vi "motor follow.vi"() -> ()   [LabVIEW 2009]
uses:
  <vilib>/NXT/Block Support/NXT_OutputPort.ctl
panel:
  in  "coeffecients":cluster{"P":dbl, "I":dbl, "D":dbl}={"P"=1.8, "I"=4.32, "D"=0.0}
  # "critical gain is around 30\noscillation period 60/130"
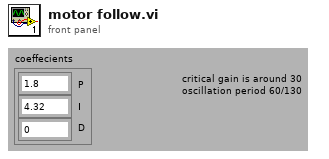
[diagram p1: front panel]
types:
  T1 = typedef "NXT_OutputPort.ctl" = u8
  T2 = typedef "SequenceBoolean.ctl" = bool
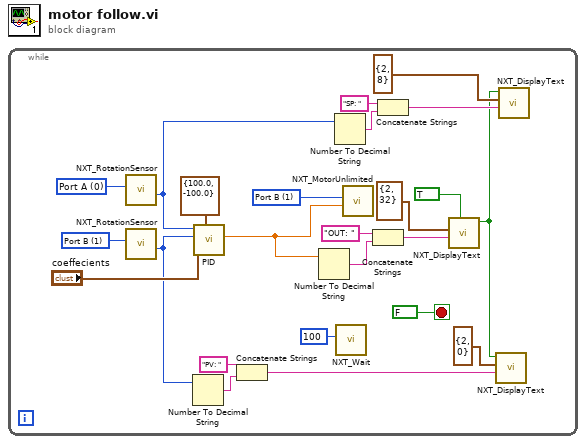
[diagram p0: block diagram]
diagram:
  n1 = while {
    stop <- FALSE stop-if-true
    w22 = T1 1 items=["Port A", "Port B", "Port C"] ("Output (Port A)")
    w23 = T1 1 items=["Port A", "Port B", "Port C"] ("Output (Port A)")
    w24 = T1 0 items=["Port A", "Port B", "Port C"] ("Output (Port A)")
    n2 = call <vilib>:"NXT_RotationSensor.vi"("Output (Port A)"=w24) -> ("Degrees out"=w5:i32)  [unwired: 7 in, 3 out]
    n3 = call <vilib>:"NXT_RotationSensor.vi"("Output (Port A)"=w23) -> ("Degrees out"=w6:i32)  [unwired: 7 in, 3 out]
    n4 = Number To Decimal String(number=w6) -> (decimal integer string=w20:string)  [unwired: 1 in]
    n5 = call "PID.vi"("range"=cluster{"max":dbl, "min":dbl} {"max"=100.0, "min"=-100.0}, "coeffecients"="coeffecients", "process variable"=w6, "setpoint"=w5) -> ("output"=w1:dbl)  [unwired: 6 in, 1 out]
    n6 = Concatenate Strings("PV: " ("string"), w20) -> (w10:string)
    n7 = Number To Decimal String(number=w1) -> (decimal integer string=w16:string)  [unwired: 1 in]
    n8 = Number To Decimal String(number=w5) -> (decimal integer string=w18:string)  [unwired: 1 in]
    n9 = call <vilib>:"NXT_Wait.vi"("Wait (ms)"=u32 100) -> ()  [unwired: 9 in, 2 out]
    n10 = call <vilib>:"NXT_MotorUnlimited.vi"("Power (75)"=w1, "Output (Port A)"=w22) -> ()  [unwired: 8 in, 2 out]
    n11 = Concatenate Strings("OUT: " ("string"), w16) -> (w12:string)
    n12 = Concatenate Strings("SP: " ("string"), w18) -> (w14:string)
    n13 = call <vilib>:"NXT_DisplayText.vi"("Clear Display (F)"=TRUE, "Text"=w12, "Location (0,0)"=cluster{"X":i16, "Y":i16} {"X"=2, "Y"=32}) -> ("Sequence Flow out"=w3:T2)  [unwired: 8 in]
    n14 = call <vilib>:"NXT_DisplayText.vi"("Text"=w10, "Location (0,0)"=cluster{"X":i16, "Y":i16} {"X"=2, "Y"=0}, "Sequence Flow in"=w3) -> ()  [unwired: 8 in, 1 out]
    n15 = call <vilib>:"NXT_DisplayText.vi"("Text"=w14, "Location (0,0)"=cluster{"X":i16, "Y":i16} {"X"=2, "Y"=8}, "Sequence Flow in"=w3) -> ()  [unwired: 8 in, 1 out]
  }
